vi "Addition&Subtraction_2NumericalValue.vi"() -> ()   [LabVIEW 2024]
panel:
  in  "Boolean":bool
  in  "milliseconds to wait":u32
  in  "stop":bool
  out "Numeric 3":dbl
  in  "Numeric 2":dbl
  in  "Numeric":dbl
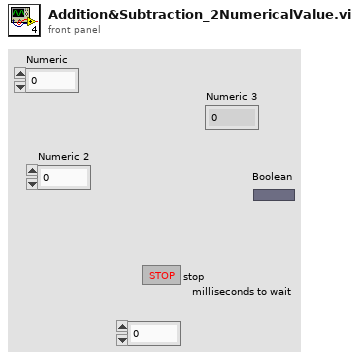
[diagram p1: front panel]
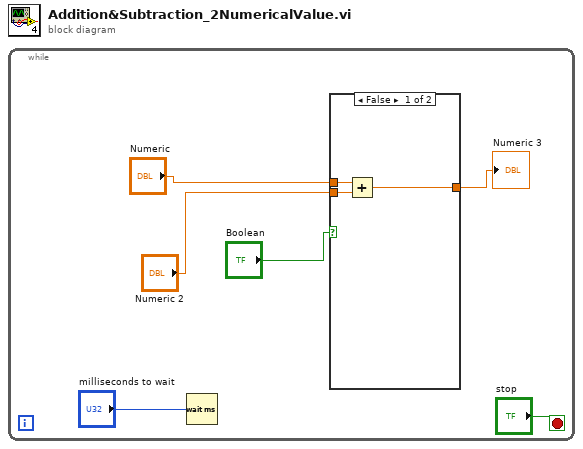
[diagram p0: block diagram]
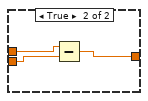
[diagram p2: hidden frame]
diagram:
  n1 = while {
    stop <- "stop" stop-if-true
    n2 = Wait (ms)(milliseconds to wait="milliseconds to wait") -> ()  [unwired: 1 out]
    n3 = case shown="False" "Boolean" {
      tunnel: "Numeric 2" -> [w9 w11]
      tunnel: "Numeric" -> [w8 w12]
      tunnel: [w7 w10] -> w2
      frame False {
        n4 = Add(x=w8, y=w9) -> (x+y=w7:dbl)
      }
      frame True {
        n5 = Subtract(x=w12, y=w11) -> (x-y=w10:dbl)
      }
    }
    "Numeric 3" <- w2
  }
